vi "Pfeiffer Vacuum Turbo access control.vi"(8 "error in (no error)":errorcluster, 9 "PV access control - Cluster":T1={"Parameter"=enum."access request", "Parameter\nread only<->describe"=FALSE, "access locked\nreleased           locked "=TRUE, "access request"=2} {"access request" items=["--", "remote", "RS 485", "--", "PV.can", "--", "--", "--", "fieldbus"]}, 10 "Adress of unit":u16=1 min=1 max=999 step=1, 11 "COM Port Name in":refnum<visa-resource-name>="COM1") -> (0 "error out":errorcluster, 3 "response (data)":string)   [LabVIEW 2016]
doc: "This VI is an example of how to use the Pfeiffer Vacuum subVIs programmatically. This VI first initializes the instrument, takes measurements, then closes the instrument."
uses:
  Public/Turbopumps/PV access control - Cluster.ctl
  Pfeiffer Vacuum.lvlib
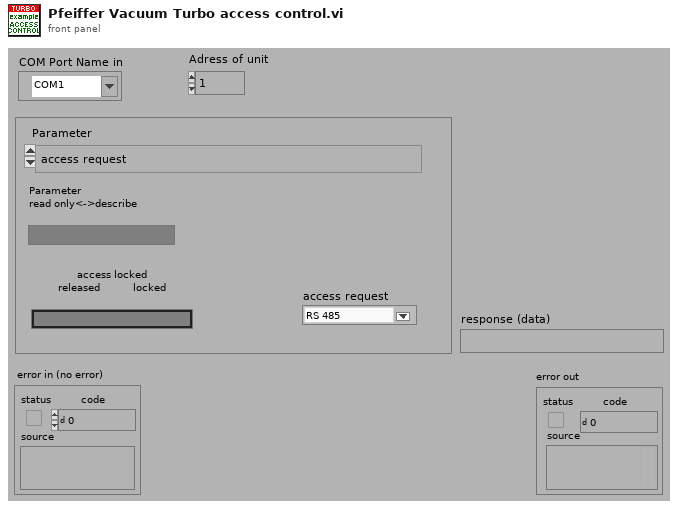
[diagram p1: front panel]
types:
  T1 = typedef "Pfeiffer Vacuum.lvlib/PV access control - Cluster.ctl" = cluster{"Parameter":enum16{"access request", "access locked"}, "Parameter\nread only<->describe":bool, "access locked\nreleased           locked ":bool, "access request":u16}
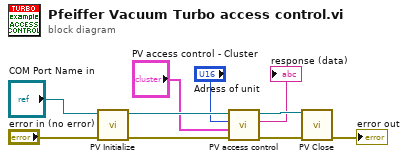
[diagram p0: block diagram]
diagram:
  n1 = call "PV Initialize.vi"("error in (no error)"="error in (no error)", "VISA session in"="COM Port Name in") -> ("error out"=w10:errorcluster, "VISA session out"=w8:refnum<visa-resource-name>)  [unwired: 8 in]
  n2 = call "PV access control.vi"("error in (no error)"=w10, "PV access control - Cluster"="PV access control - Cluster", "Adress of unit"="Adress of unit", "VISA session"=w8) -> ("error out"=w9:errorcluster, "response (data)"=→"response (data)":string, "dup VISA session"=w7:refnum<visa-resource-name>)  [unwired: 4 in]
  n3 = call "PV Close.vi"("VISA session"=w7, "error in (no error)"=w9) -> ("error out"=→"error out":errorcluster)  [unwired: 13 in]
